vi "Save Rx Data.vi"(11 "Buffer in":u8[](array[numeric])) -> ()   [LabVIEW 2015]
uses:
  <vilib>/Utility/sysdir.llb/System Directory Type.ctl
  <vilib>/Utility/file.llb/Write To Spreadsheet File (I64).vi
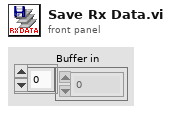
[diagram p1: front panel]
types:
  T1 = typedef "System Directory Type.ctl" = i32
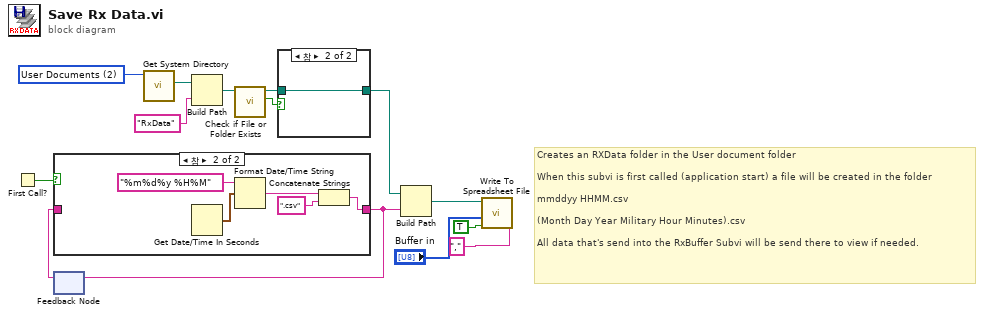
[diagram p0: block diagram]
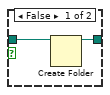
[diagram p3: hidden frame]
diagram:
  w12 = T1 2 items=["User Home"=0, "User Desktop"=1, "User Documents"=2, "User Application Data"=3, "User Preferences"=4, "User Temporary"=5, "Public Documents"=6, "Public Application Data"=7, "Public Preferences"=8, "Public Cache"=13, "System Core Libraries"=9, "System Installed Libraries"=10, "Application Files"=11, "Boot Volume Root"=12] ("system directory type")
  # "Creates an RXData folder in the User document folder\n\nWhen this subvi is first called (application start) a file will be created in the folder\n\nmmddyy HHMM.csv\n\n(Month Day Year Military Hour Minutes).csv\n\nAll data that's send into the RxBuffer Subvi will be send there to view if needed."
  n1 = First Call?() -> (First Call?: T/F=w3:bool)
  n2 = feedback #1() -> (w1:string)  [unwired: 1 in]
  n3 = case shown="참" w3 {
    tunnel: [w15 w16] -> w2
    tunnel: w1 -> [w15 _]
    frame False {
    }
    frame True {
      n4 = Get Date/Time In Seconds() -> (seconds since 1Jan1904=w20:timestamp)
      n5 = Format Date/Time String(time format string (%c)="%m%d%y %H%M", seconds (now)=w20) -> (date/time string=w18:string)  [unwired: 1 in]
      n6 = Concatenate Strings(w18, ".csv" ("string")) -> (w16:string)
    }
  }
  n7 = feedback-in #1(w2) -> ()
  n8 = call <vilib>:"Get System Directory.vi"("system directory type"=w12) -> ("system directory"=w9:path)  [unwired: 10 in]
  n9 = Build Path(base path=w9, name or relative path="RxData") -> (appended path=w7:path)
  n10 = call <vilib>:"Check if File or Folder Exists.vi"("path"=w7) -> ("file or folder exists?"=w6:bool, "dup path"=w5:path)  [unwired: 8 in, 1 out]
  n11 = case shown="참" w6 {
    tunnel: w5 -> [w22 w23]
    tunnel: [w21 w23] -> w4
    frame False {
      n12 = Create Folder(path (use dialog)=w22) -> (created path=w21:path)  [unwired: 2 in, 2 out]
    }
    frame True {
    }
  }
  n13 = Build Path(base path=w4, name or relative path=w2) -> (appended path=w11:path)
  n14 = call-poly <vilib>:"Write To Spreadsheet File.vi"("delimiter (\\t)"="," ("delimiter (\\t)"), "append to file? (new file:F)"=TRUE, "1D data"="Buffer in", "file path (dialog if empty)"=w11) -> ()  [unwired: 4 in, 1 out]
